vi "1.1 Lead For Steering.vi"(0 "Input K s14fxp-6":fxp<+/-,14,-6> format="%.19g", 1 "Input C u8fxp-2":fxp<+,8,-2>, 2 "Error Input":i32) -> (3 "s(sqrt(10)s+bdt)/(s/sqrt(10)+bdt)":fxp<+/-,20,22>, 4 "(sqrt(10)s+bdt)/(s/sqrt(10)+bdt)":fxp<+/-,20,22>, 5 "sqrt(10)s+bdt":fxp<+/-,18,20>, 6 "Controls Output":fxp<+/-,20,5> format="%.17g")   [LabVIEW 2011]
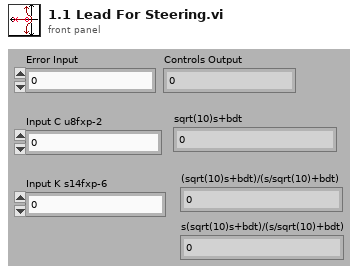
[diagram p1: front panel]
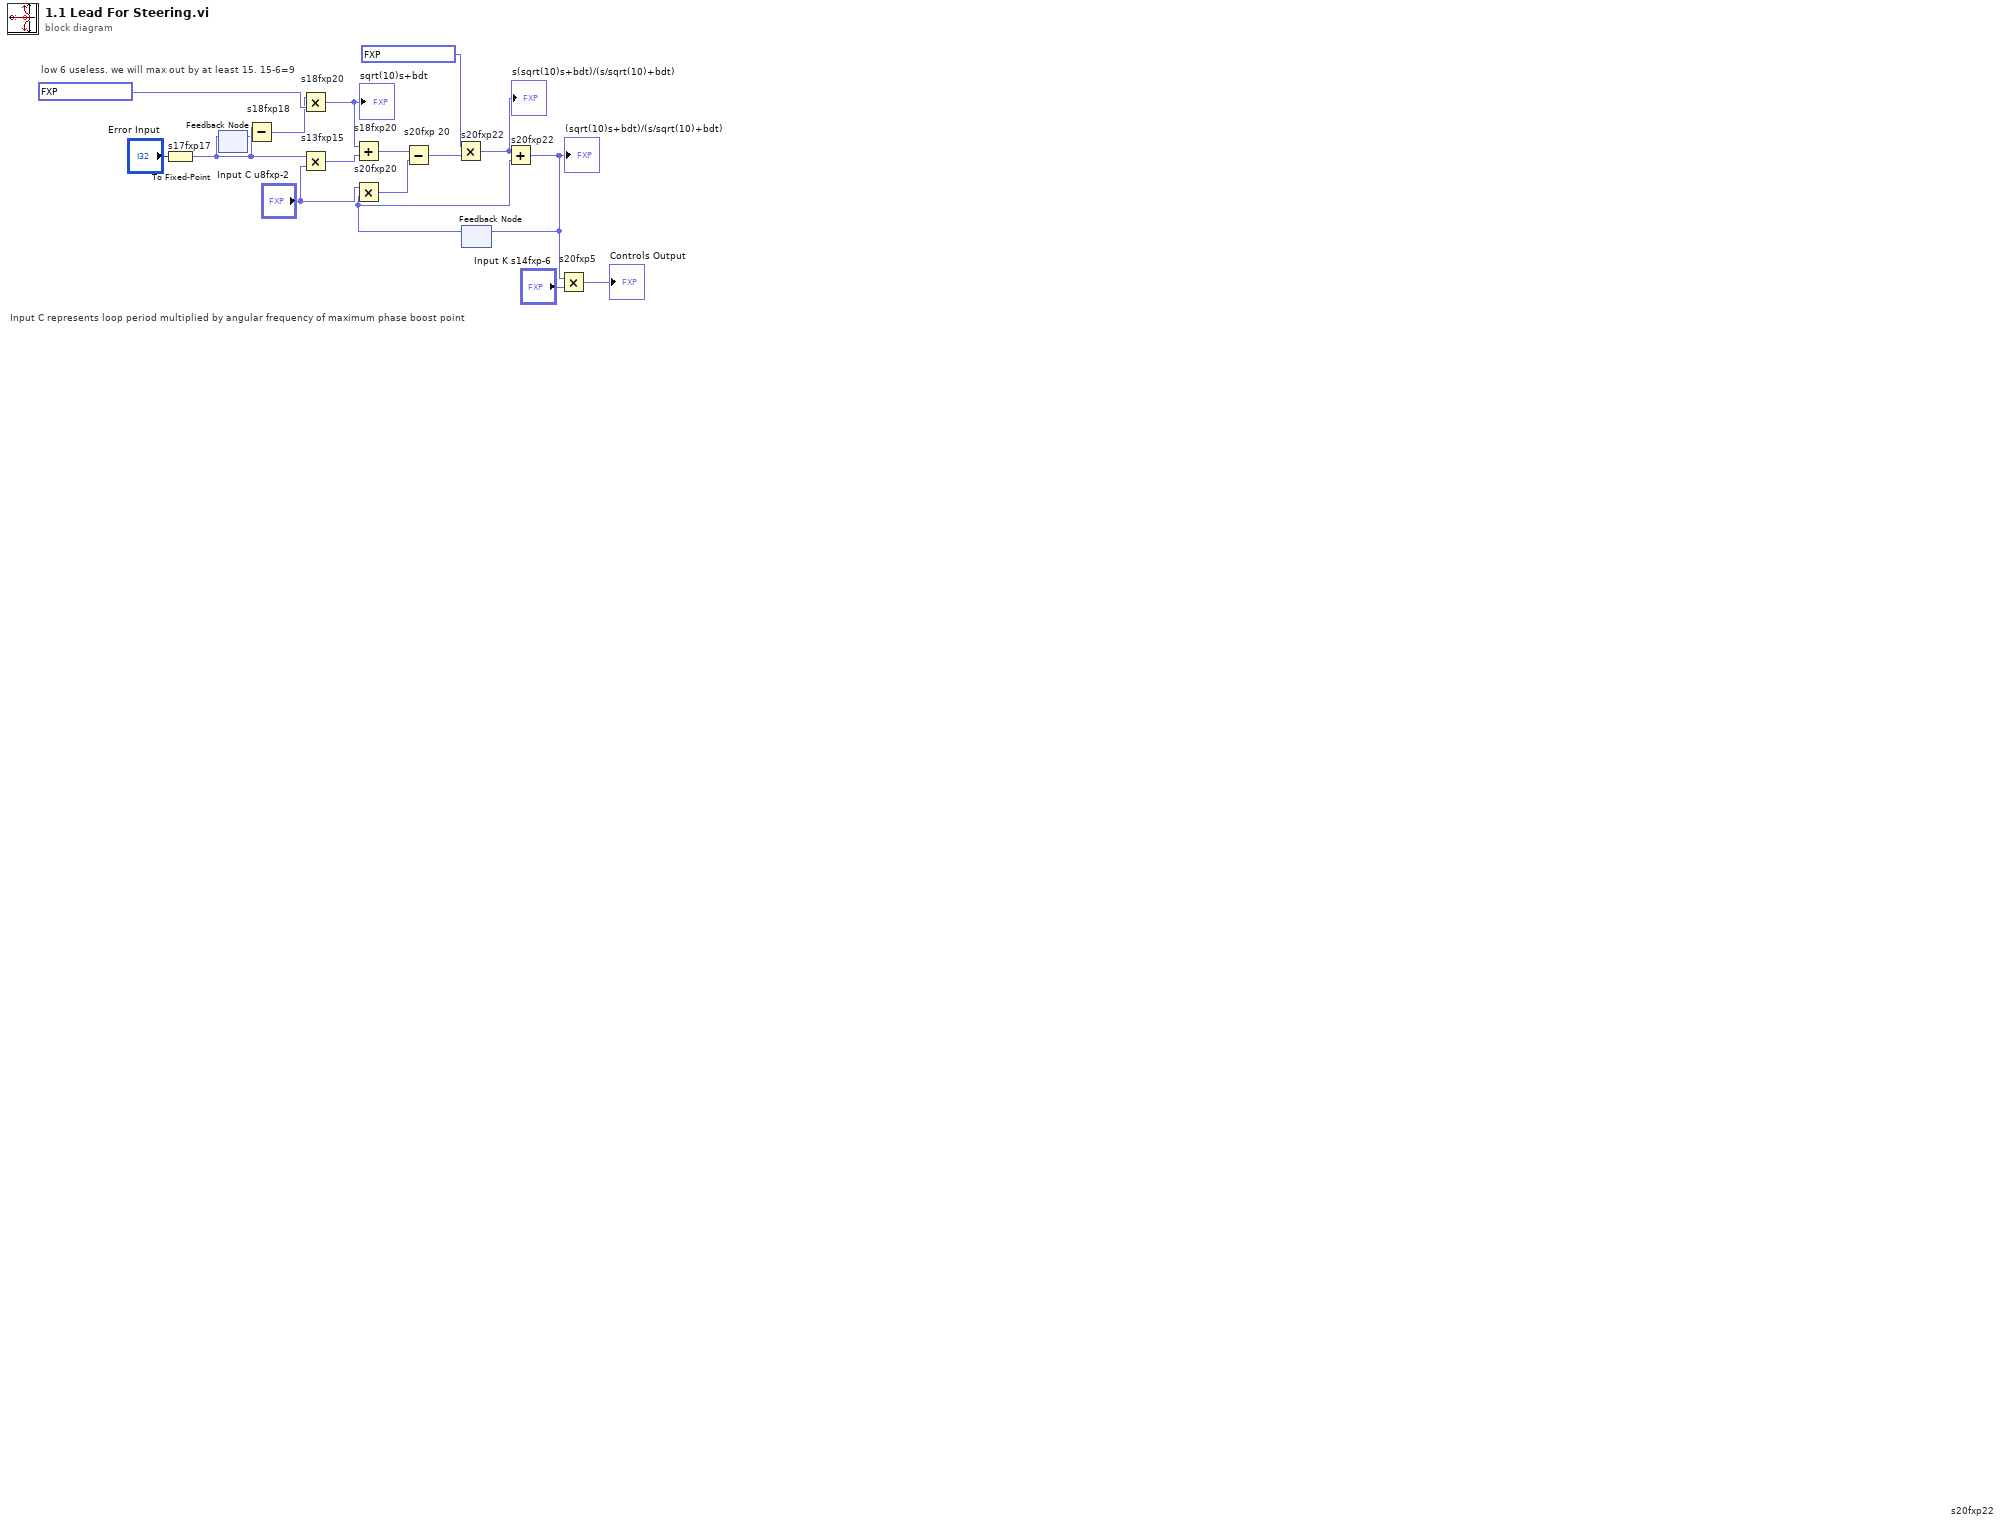
[diagram p0: block diagram]
diagram:
  # "low 6 useless. we will max out by at least 15. 15-6=9"
  # "Input C represents loop period multiplied by angular frequency of maximum phase boost point"
  n1 = To Fixed-Point "s17fxp17"(number="Error Input") -> (fixed-point=w5:fxp<+/-,17,17>)  [unwired: 1 in]
  n2 = feedback #1() -> (w1:fxp<+/-,17,17>)  [unwired: 1 in]
  n3 = feedback-in #1(w5) -> ()
  n4 = Subtract "s18fxp18"(x=w5, y=w1) -> (x-y=w2:fxp<+/-,18,18>)
  n5 = Multiply "s18fxp20"(x=w2, y=fxp<+/-,18,3> 3.16229248046875) -> (x*y=w4:fxp<+/-,18,20>)
  "sqrt(10)s+bdt" <- w4
  n6 = Multiply "s13fxp15"(x=w5, y="Input C u8fxp-2") -> (x*y=w6:fxp<+/-,13,15>)
  n7 = Add "s18fxp20"(x=w4, y=w6) -> (x+y=w8:fxp<+/-,18,20>)
  n8 = feedback #2 "s20fxp22"() -> (w13:fxp<+/-,20,22>)  [unwired: 1 in]
  n9 = Multiply "s20fxp20"(x="Input C u8fxp-2", y=w13) -> (x*y=w9:fxp<+/-,20,20>)
  n10 = Subtract "s20fxp 20"(x=w8, y=w9) -> (x-y=w10:fxp<+/-,20,20>)
  n11 = Multiply "s20fxp22"(x=fxp<+/-,18,3> 3.16229248046875 ("y"), y=w10) -> (x*y=w12:fxp<+/-,20,22>)
  "s(sqrt(10)s+bdt)/(s/sqrt(10)+bdt)" <- w12
  n12 = Add "s20fxp22"(x=w12, y=w13) -> (x+y=w14:fxp<+/-,20,22>)
  "(sqrt(10)s+bdt)/(s/sqrt(10)+bdt)" <- w14
  n13 = feedback-in #2(w14) -> ()
  n14 = Multiply "s20fxp5"(x=w14, y="Input K s14fxp-6") -> (x*y=→"Controls Output":fxp<+/-,20,5>)
